vi "FRC Timer 3.vi"(8 "Error In":errorcluster, 10 "Time Target (s)":dbl=4.0, 11 "Boolean":bool) -> (0 "Error Out":errorcluster, 2 "Has Time Elapsed":bool, 3 "Elapsed Time (s.ms)":dbl format="%#.2f")   [LabVIEW 2016]
doc: "CLD 3 Exercise\nThis VI is used as a timer functional global. \nNote on reading time when in pause. The developer should not call the read time function when in pause; however, a case structure is used to defensively program the read state for this possibility."
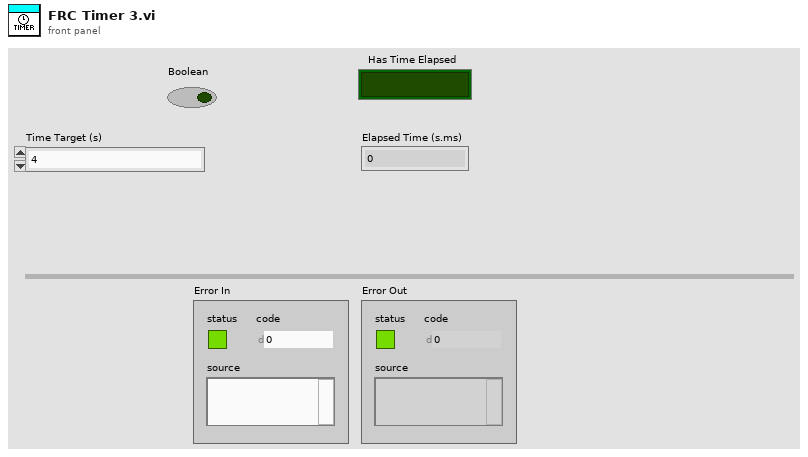
[diagram p1: front panel]
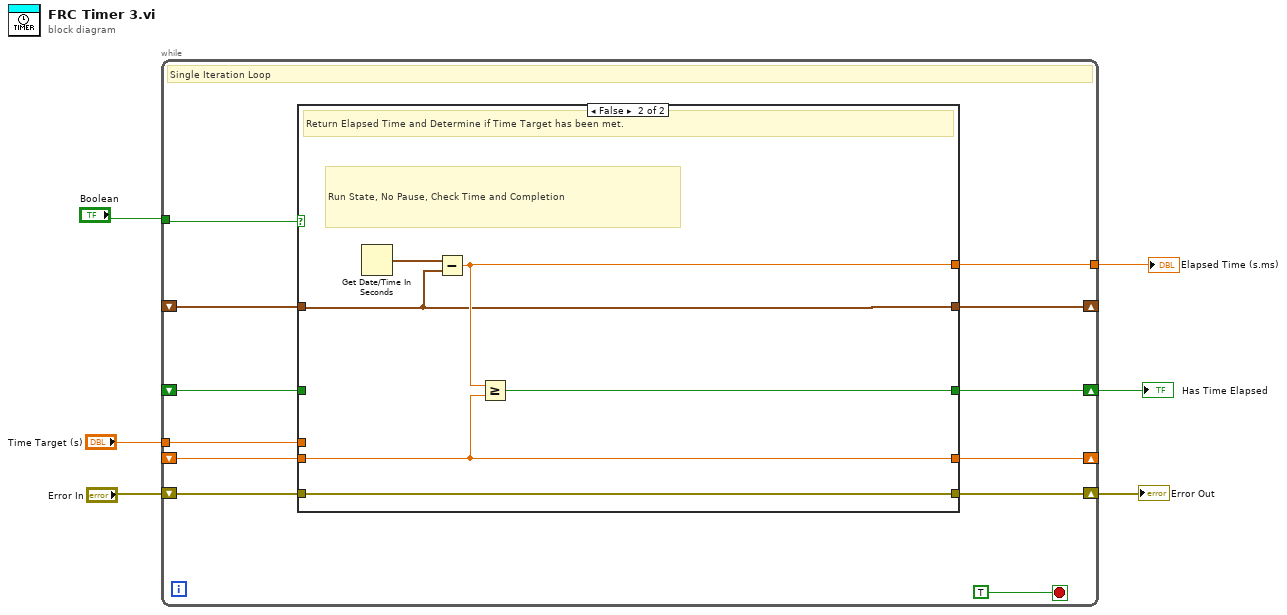
[diagram p0: block diagram]
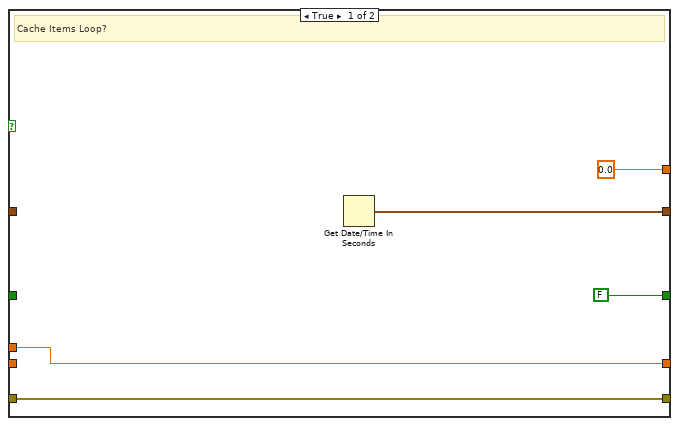
[diagram p2: hidden frame]
diagram:
  n1 = while {
    shift-right: [w17] -> _
    shift-left: _ -> [w16]
    tunnel: [w15] -> w2
    shift-right: [w14] -> w6
    shift-left: "Error In" -> [w13]
    tunnel: "Time Target (s)" -> [w10]
    shift-right: [w11] -> _
    shift-left: _ -> [w12]
    shift-right: [w9] -> w3
    shift-left: _ -> [w8]
    tunnel: "Boolean" -> [w7]
    stop <- TRUE ("stop") stop-if-true
    # "Single Iteration Loop"
    n2 = case shown="False" w7 {
      tunnel: [w23 w25] -> w17
      tunnel: w16 -> [_ w25]
      tunnel: [0.0 ("Elapsed Time") w26] -> w15
      tunnel: [w21 w29] -> w14
      tunnel: w13 -> [w21 w29]
      tunnel: w12 -> [_ w28]
      tunnel: [w20 w28] -> w11
      tunnel: w10 -> [w20 _]
      tunnel: [FALSE w27] -> w9
      tunnel: w8 -> [_ _]
      frame True {
        # "Cache Items Loop?"
        n3 = Get Date/Time In Seconds() -> (seconds since 1Jan1904=w23:timestamp)
      }
      frame False {
        # "Run State, No Pause, Check Time and Completion"
        # "Return Elapsed Time and Determine if Time Target has been met."
        n4 = Get Date/Time In Seconds() -> (seconds since 1Jan1904=w24:timestamp)
        n5 = Subtract(x=w24, y=w25) -> (x-y=w26:dbl)
        n6 = Greater Or Equal?(x=w26, y=w28) -> (x >= y?=w27:bool)
      }
    }
  }
  "Error Out" <- w6
  "Has Time Elapsed" <- w3
  "Elapsed Time (s.ms)" <- w2
